vi "PID control XY vel.vi"() -> ()   [LabVIEW 2010]
uses:
  <vilib>/addons/control/pid/pid.llb/PID (DBL Array).vi
  <vilib>/addons/control/pid/NI_PID_pid.lvlib
panel:
  out "z pos /100 nm":dbl
  out "y vel (mm/s)":dbl
  out "x vel (mm/s)":dbl
  in  "reinitialize? (F)":bool
  in  "z position range (um)":cluster{"output high":dbl, "output low":dbl}={"output high"=2.0, "output low"=-2.0} {"output low" format="%.2f"; "output high" format="%.2f"}
  in  "z polarity":bool
  in  "y polarity":bool
  in  "x polarity":bool
  in  "z location (um)":dbl
  in  "Z gains":T1={"proportional gain (Kc)"=1.0, "integral time (Ti, min)"=0.01, "derivative time (Td, min)"=0.0} {"derivative time (Td, min)" format="%.3f"; "integral time (Ti, min)" format="%.3f"; "proportional gain (Kc)" format="%.3f"}
  in  "XY gains":T2={"chase time (ms)"=200.0, "integral time (Ti, sec)"=0.001, "derivative time (Td, sec)"=0.0} {"derivative time (Td, sec)" format="%.3f"; "integral time (Ti, sec)" format="%.3f"; "chase time (ms)" format="%.3f"}
  in  "XY vel range (mm/s)":cluster{"output high":dbl, "output low":dbl}={"output high"=2.0, "output low"=-2.0} {"output low" format="%.2f"; "output high" format="%.2f"}
  in  "measurement time":dbl
  in  "y location (um)":dbl
  in  "x location (um)":dbl
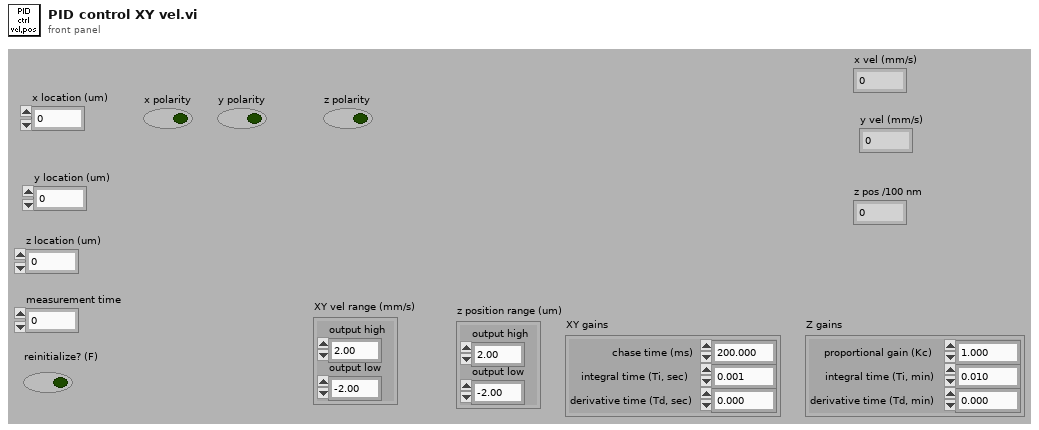
[diagram p1: front panel]
types:
  T1 = cluster{"proportional gain (Kc)":dbl, "integral time (Ti, min)":dbl, "derivative time (Td, min)":dbl}
  T2 = cluster{"chase time (ms)":dbl, "integral time (Ti, sec)":dbl, "derivative time (Td, sec)":dbl}
  T3 = cluster{"proportional gain (Kc)":dbl, "integral time (Ti, min)":dbl, "derivative time (Td, min)":dbl}[]
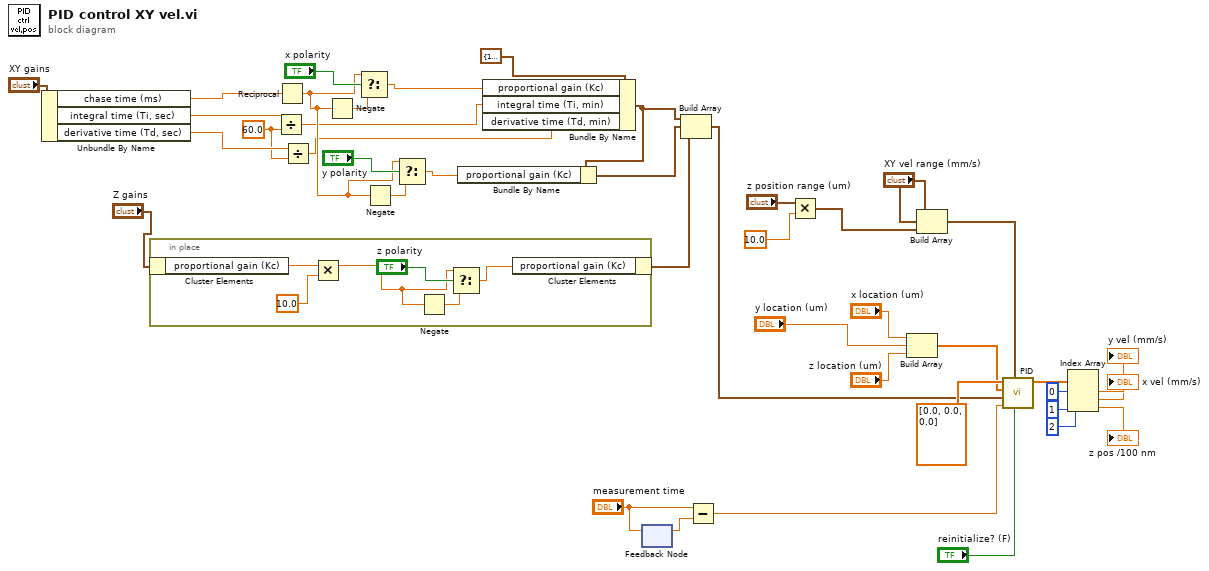
[diagram p0: block diagram]
diagram:
  w34 = 60.0 ("y")
  n1 = Unbundle By Name("XY gains") -> ("chase time (ms)"=w33:dbl, "integral time (Ti, sec)"=w36:dbl, "derivative time (Td, sec)"=w35:dbl)
  n2 = in-place {
    n3 = in-place-cluster #1("Z gains") -> ("proportional gain (Kc)"=w45:dbl)
    n4 = Multiply(x=w45, y=10.0) -> (x*y=w43:dbl)
    n5 = Negate(x=w43) -> (-x=w46:dbl)
    n6 = Select(t=w43, s="z polarity", f=w46) -> (s? t:f=w44:dbl)
    n7 = in-place-cluster #1("proportional gain (Kc)"=w44) -> (w19:T1)
  }
  n8 = Divide(x=w36, y=w34) -> (x/y=w26:dbl)
  n9 = Reciprocal(x=w33) -> (1/x=w28:dbl)
  n10 = Divide(x=w35, y=w34) -> (x/y=w25:dbl)
  n11 = Negate(x=w28) -> (-x=w31:dbl)
  n12 = Select(t=w28, s="x polarity", f=w31) -> (s? t:f=w27:dbl)
  n13 = Negate(x=w28) -> (-x=w29:dbl)
  n14 = Select(t=w28, s="y polarity", f=w29) -> (s? t:f=w23:dbl)
  n15 = Bundle By Name(cluster=T1 {"proportional gain (Kc)"=1.0, "integral time (Ti, min)"=0.01, "derivative time (Td, min)"=0.0} ("Z gains"), "proportional gain (Kc)"=w27, "integral time (Ti, min)"=w26, "derivative time (Td, min)"=w25) -> (w22:T1)
  n16 = Bundle By Name(cluster=w22, "proportional gain (Kc)"=w23) -> (w21:T1)
  n17 = feedback-in #2("measurement time") -> ()
  n18 = feedback #2() -> (w39:dbl)  [unwired: 1 in]
  n19 = Build Array(w22, w21, w19) -> (w18:T3)
  n20 = Subtract(x="measurement time", y=w39) -> (x-y=w38:dbl)
  n21 = Multiply(x="z position range (um)", y=10.0 ("measurement time")) -> (x*y=w11:cluster{"output high":dbl, "output low":dbl})
  n22 = Build Array("x location (um)", "y location (um)", "z location (um)") -> (w10:dbl[])
  n23 = Build Array("XY vel range (mm/s)", "XY vel range (mm/s)", w11) -> (w9:cluster{"output high":dbl, "output low":dbl}[])
  n24 = call-poly <vilib>:"PID.vi"("reinitialize? (F)"="reinitialize? (F)", "output range"=w9, "dt (s)"=w38, "PID gains"=w18, "process variable"=w10, "setpoint"=dbl[] [0.0, 0.0, 0.0]) -> ("output"=w7:dbl[])  [unwired: 4 in, 1 out]
  n25 = Index Array(array=w7, index #1=0 ("index"), index #2=1 ("index"), index #3=2 ("index")) -> (element #1=→"x vel (mm/s)":dbl, element #2=→"y vel (mm/s)":dbl, element #3=→"z pos /100 nm":dbl)
